vi "Get Data Out.vi"(8 "error in (no error)":errorcluster) -> (0 "error out":errorcluster, 3 "DataOut":T1)   [LabVIEW 2017]
doc: "This VI reads the outbound data from the 'All data' FGV"
uses:
  TypeDefs/dataOut.ctl
  FGVs/TypeDefs/DataFGVControl.ctl
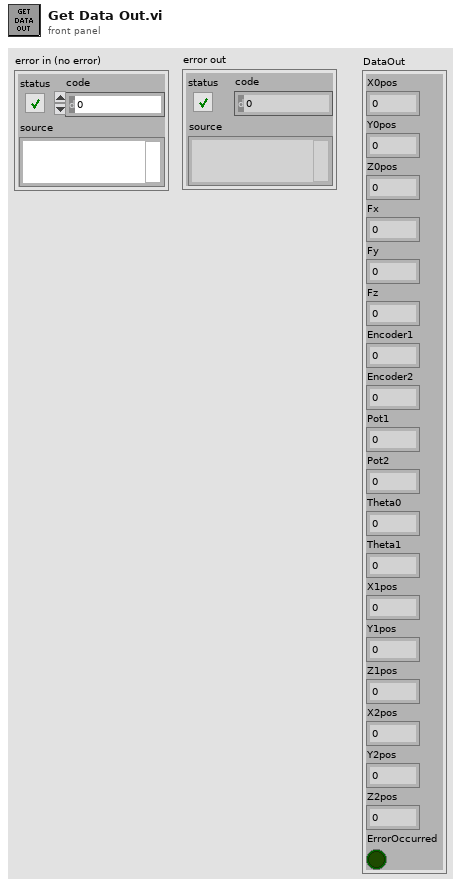
[diagram p1: front panel]
types:
  T1 = typedef "dataOut.ctl" = cluster{"X0pos":dbl, "Y0pos":dbl, "Z0pos":dbl, "Fx":dbl, "Fy":dbl, "Fz":dbl, "Encoder1":i32, "Encoder2":i32, "Pot1":dbl, "Pot2":dbl, "Theta0":dbl, "Theta1":dbl, "X1pos":dbl, "Y1pos":dbl, "Z1pos":dbl, "X2pos":dbl, "Y2pos":dbl, "Z2pos":dbl, "ErrorOccurred":bool}
  T2 = typedef "DataFGVControl.ctl" = enum16{"Set Data", "Get Data"}
  T3 = typedef "allData.ctl" = cluster{"DataOut":T1, "DataIn":T4}
  T4 = typedef "dataIn.ctl" = cluster{"Xtarget":dbl, "Ytarget":dbl, "Ztarget":dbl, "X_Attractor1":dbl, "Y_Attractor1":dbl, "Z_Attractor1":dbl, "X_Attractor2":dbl, "Y_Attractor2":dbl, "Z_Attractor2":dbl, "Traj_Flag":bool, "DeadZone":dbl, "Assistance":bool, "Shutdown":bool, "AssistanceLevel":dbl}
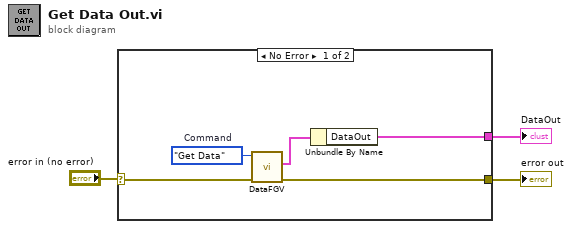
[diagram p0: block diagram]
diagram:
  n1 = case shown="No Error" "error in (no error)" {
    selector: "error in (no error)" -> [w8 w9]
    tunnel: [w7 w9] -> w2
    tunnel: [w4 _] -> w1
    frame No Error {
      w6 = DataFGVControl."Get Data"  # Command
      n2 = call "DataFGV.vi"("error in (no error)"=w8, "Command"=w6) -> ("error out"=w7:errorcluster, "AllData out"=w5:T3)  [unwired: 8 in]
      n3 = Unbundle By Name(w5) -> ("DataOut"=w4:T1)
    }
    frame Error {
    }
  }
  "error out" <- w2
  "DataOut" <- w1
